vi "initialize.vi"(0 "HGF_Factory":refnum<class "HGF_Factory.lvclass">, 3 "initializationData":variant, 5 "error in (no error)":errorcluster, 7 "binaryString":string, 8 "I8 Array":i8[](array[numeric]), 9 "prependSize? (T)":bool, 11 "byteOrder (0:big-endian, network order)":T1(ring)) -> (14 "dup HGF_Factory":refnum<class "HGF_Factory.lvclass">, 17 "found?":bool, 19 "error out":errorcluster)   [LabVIEW 2014, in "HGF_BaseClasses.lvlib" / "HGF_Factory.lvclass"]
doc: "This is a dynamic dispatch VI to be implemented by child classes to initialize their attributes.\n\n<B>Recommendation:</B> Use Variant for initialization data."
uses:
  HGF_Factory.lvclass
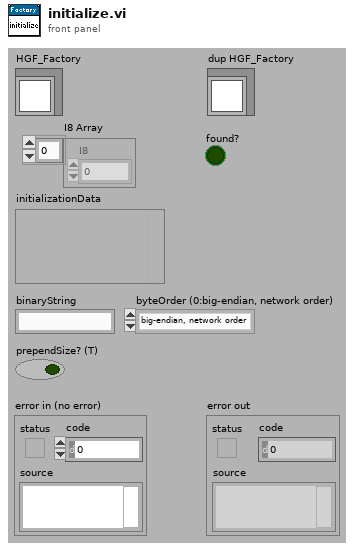
[diagram p1: front panel]
types:
  T1 = enum16{"big-endian, network order", "native, host order", "little-endian"}
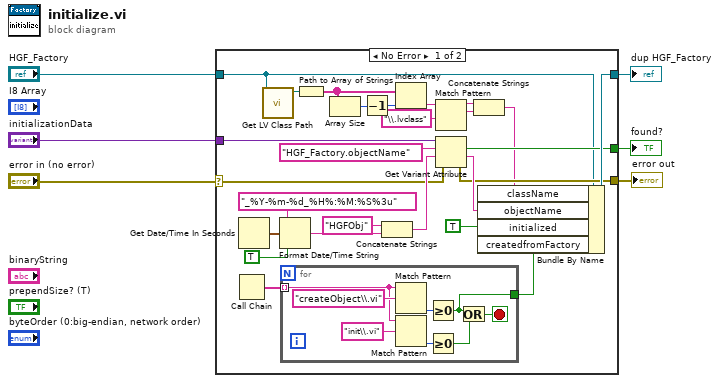
[diagram p0: block diagram]
diagram:
  n1 = case shown="No Error" "error in (no error)" {
    selector: "error in (no error)" -> [w15 w42]
    tunnel: [w14 w42] -> w5
    tunnel: [w31 w41] -> w3
    tunnel: "HGF_Factory" -> [w9 w41]
    tunnel: "initializationData" -> [w24 _]
    tunnel: [w16 _] -> w1
    frame No Error {
      n2 = Call Chain() -> (call chain=w32:string[])
      n3 = Get Date/Time In Seconds() -> (seconds since 1Jan1904=w19:timestamp)
      n4 = call <vilib>:"Get LV Class Path.vi"("object"=w9) -> ("class path"=w13:path)  [unwired: 1 in, 9 out]
      n5 = Format Date/Time String(time format string (%c)="_%Y-%m-%d_%H%:%M:%S%3u", seconds (now)=w19, UTC format=TRUE) -> (date/time string=w22:string)
      n6 = for {
        tunnel: w32 -> [w36] mode=indexing
        tunnel: [w33] -> w30
        stop <- w34 stop-if-true
        n7 = Match Pattern(string=w36, regular expression="createObject\\.vi") -> (offset past match=w40:i32)  [unwired: 4 out]
        n8 = Match Pattern(string=w36, regular expression="init\\.vi") -> (offset past match=w39:i32)  [unwired: 4 out]
        n9 = Greater Or Equal To 0?(x=w40) -> (x >= 0?=w33:bool)
        n10 = Greater Or Equal To 0?(x=w39) -> (x >= 0?=w35:bool)
        n11 = Or(x=w33, y=w35) -> (x .or. y?=w34:bool)
      }
      n12 = Path to Array of Strings(0:w13) -> (2:w12:string[])  [unwired: 1 out]
      n13 = Array Size(array=w12) -> (size(s)=w11:i32)
      n14 = Decrement(x=w11) -> (x-1=w10:i32)
      n15 = Concatenate Strings("HGFObj" ("name"), w22) -> (w18:string)
      n16 = Index Array(array=w12, index=w10) -> (element=w8:string)
      n17 = Match Pattern(string=w8, regular expression="\\.lvclass") -> (before substring=w29:string, match substring=w28:string)  [unwired: 3 out]
      n18 = Get Variant Attribute(Variant=w24, name="HGF_Factory.objectName", default value (empty Variant)=w18, error in=w15) -> (found=w16:bool, value=w17:string, error out=w14:errorcluster)  [unwired: 1 out]
      n19 = Concatenate Strings(w29, w28) -> (w7:string)
      n20 = Bundle By Name(cluster=w9, "className"=w7, "objectName"=w17, "initialized"=TRUE, "createdfromFactory"=w30) -> (w31:refnum<class "HGF_Factory.lvclass">)
    }
    frame Error {
    }
  }
  "error out" <- w5
  "dup HGF_Factory" <- w3
  "found?" <- w1
